vi "Merge_metadata.vi"(2 "New Value Priority high?":bool, 3 "Comments Row Number":i32, 4 "New Values In":string[](array[string]), 5 "New Chs In":string[](array[string]), 6 "Orig Values In":string[][](array[string]), 7 "Orig Chs In":string[](array[string])) -> (0 "Channel Values Out":string[][](array[string]), 1 "Ch names Out":string[](array[string]))   [LabVIEW 2010]
panel:
  out "Case":string
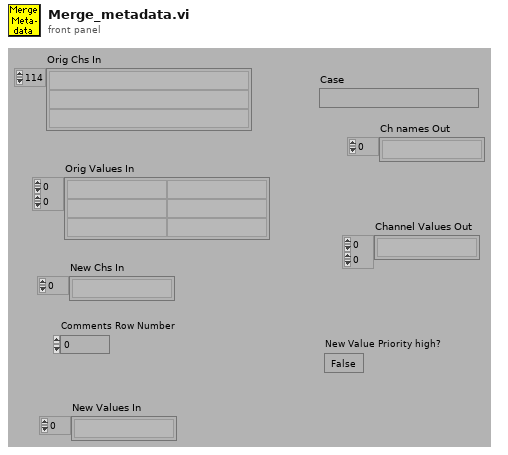
[diagram p1: front panel]
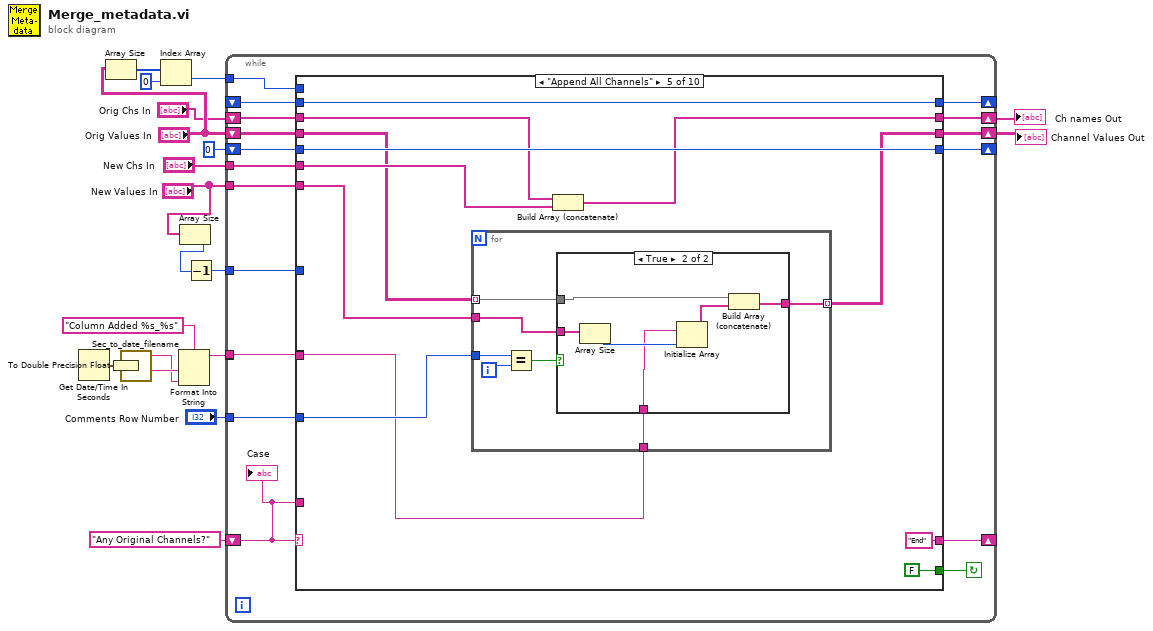
[diagram p0: block diagram]
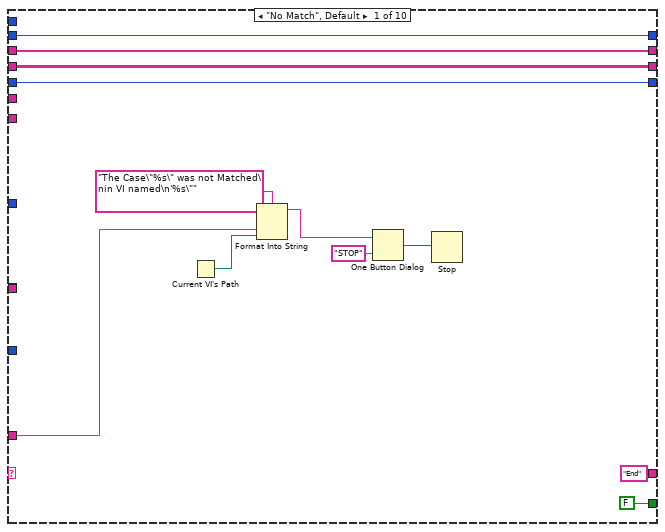
[diagram p2: hidden frame]
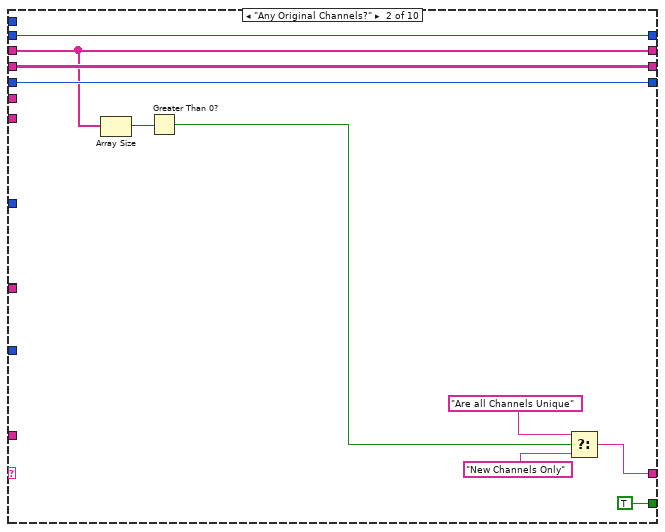
[diagram p3: hidden frame]
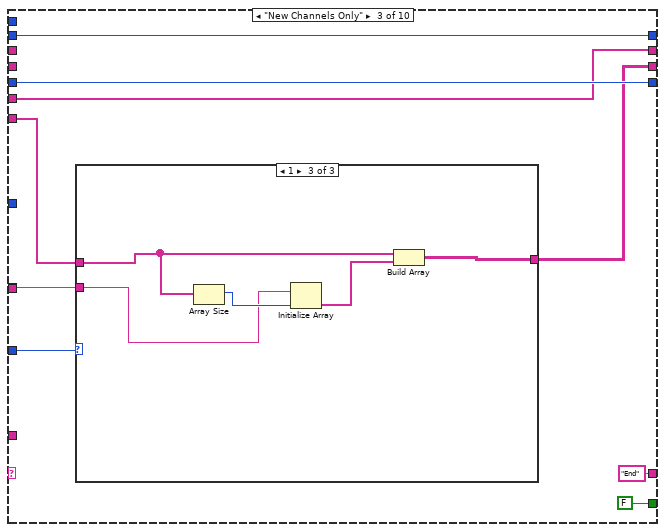
[diagram p4: hidden frame]
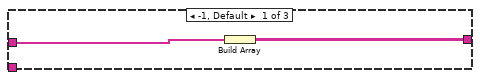
[diagram p5: hidden frame]
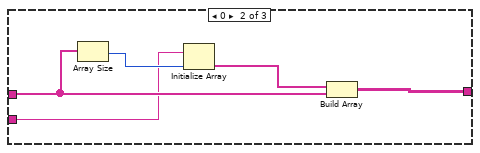
[diagram p6: hidden frame]
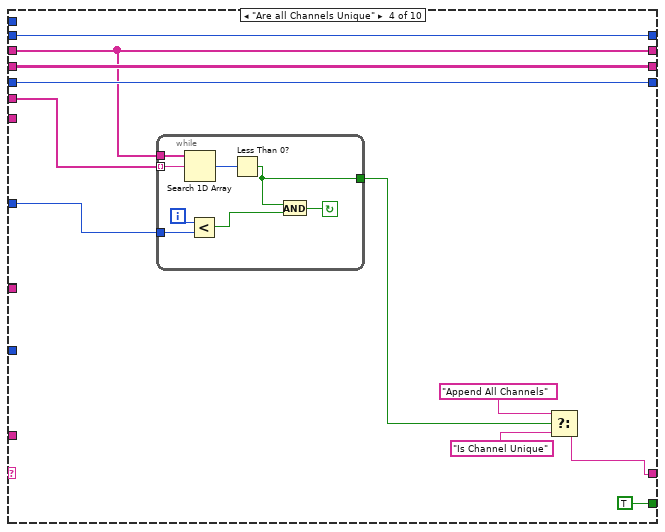
[diagram p7: hidden frame]
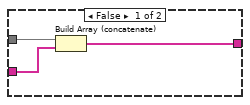
[diagram p8: hidden frame]
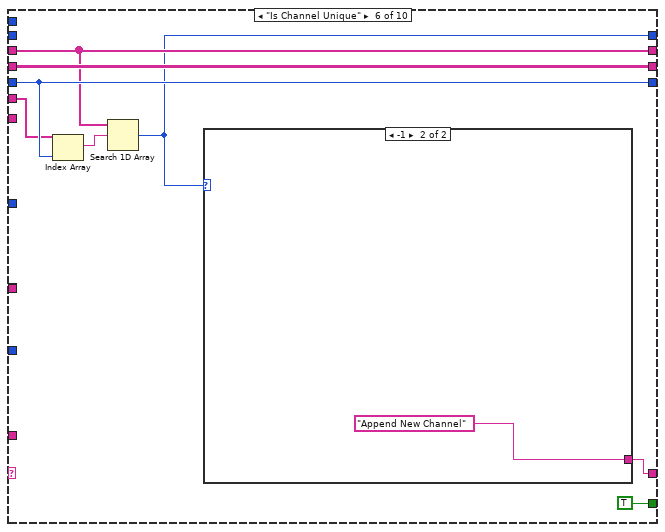
[diagram p9: hidden frame]
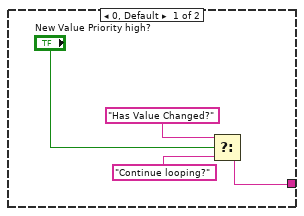
[diagram p10: hidden frame]
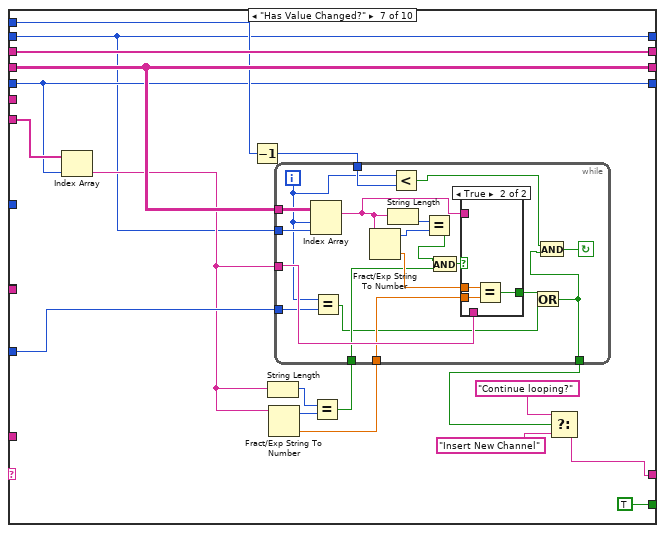
[diagram p11: hidden frame]
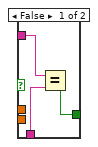
[diagram p12: hidden frame]
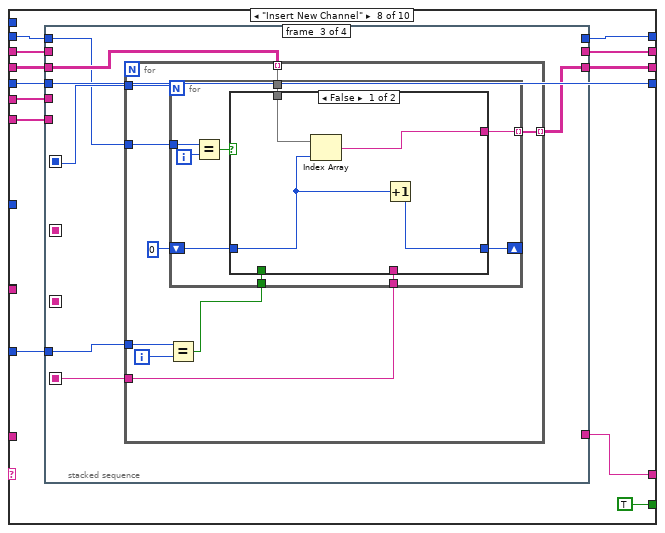
[diagram p13: hidden frame]
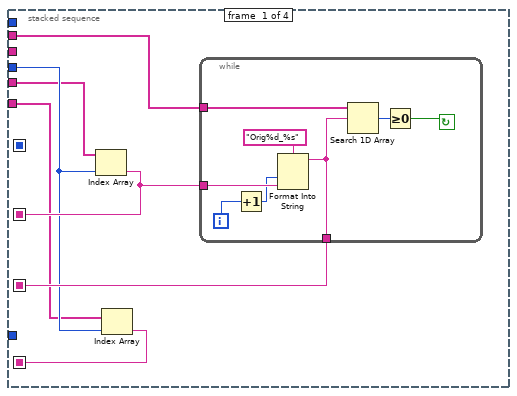
[diagram p14: hidden frame]
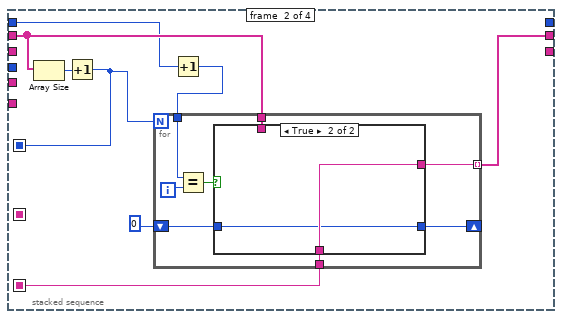
[diagram p15: hidden frame]
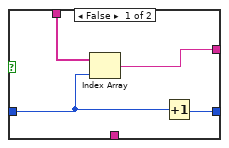
[diagram p16: hidden frame]
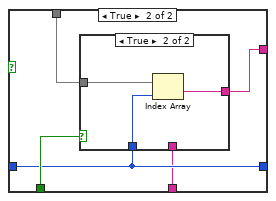
[diagram p17: hidden frame]
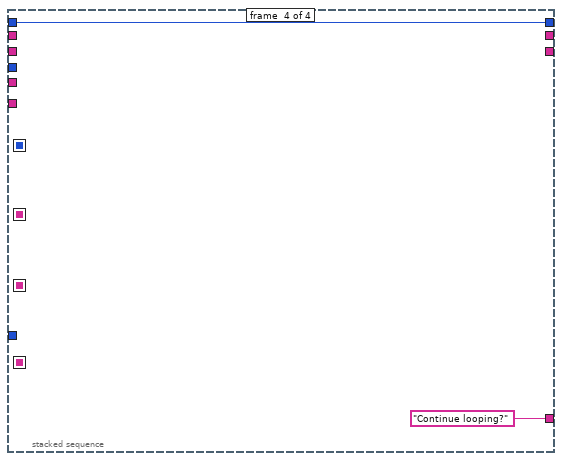
[diagram p19: hidden frame]
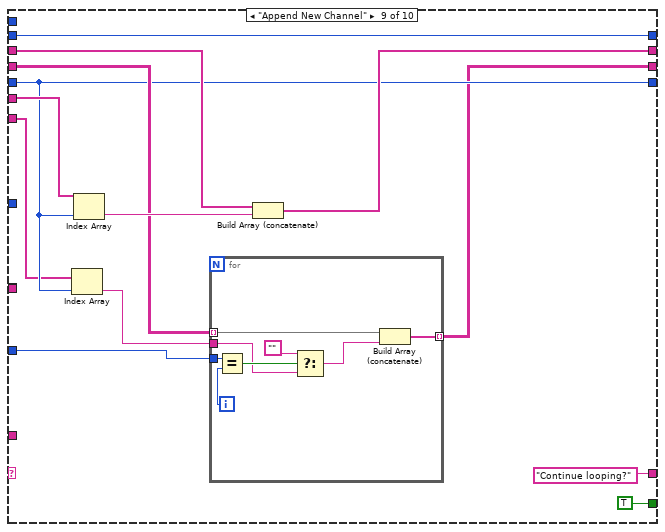
[diagram p20: hidden frame]
diagram:
  n1 = Get Date/Time In Seconds() -> (seconds since 1Jan1904=w1:timestamp)
  n2 = Array Size(array="Orig Values In") -> (size(s)=w14:i32[])
  n3 = To Double Precision Float(number=w1) -> (double precision float=w4:dbl)
  n4 = call "Sec_to_date_filename.vi"("seconds"=w4) -> ("Year"=w2:string, "Day"=w3:string)  [unwired: 2 out]
  n5 = Index Array(array=w14, index=0 ("Index")) -> (element=w11:i32)
  n6 = Format Into String(format string="Column Added %s_%s" ("Format String"), w3, w2) -> (resulting string=w5:string)  [unwired: 2 in, 1 out]
  n7 = Array Size(array="New Values In") -> (size(s)=w16:i32)
  n8 = Decrement(x=w16) -> (x-1=w15:i32)
  n9 = while {
    tunnel: w5 -> [w21]
    tunnel: w5 -> [w22]
    shift-left: _ -> [w24]
    shift-right: [w23] -> _
    tunnel: "Comments Row Number" -> [w25]
    tunnel: "New Values In" -> [w26]
    tunnel: "New Chs In" -> [w27]
    tunnel: w11 -> [w28]
    tunnel: w15 -> [w29]
    shift-left: 0 -> [w30]
    shift-right: [w31] -> _
    shift-left: "Orig Values In" -> [w33]
    shift-right: [w32] -> w18
    shift-left: "Orig Chs In" -> [w34]
    shift-right: [w35] -> w19
    shift-left: "Any Original Channels?" -> [w37]
    shift-right: [w36] -> _
    stop <- w38 continue-if-true
    n10 = case shown="\"Append All Channels\"" w37 {
      tunnel: [FALSE ("Results File?") TRUE ("Results File?") FALSE ("Results File?") TRUE ("Results File?") FALSE ("Results File?") TRUE ("Results File?") TRUE ("Results File?") TRUE ("Results File?") TRUE ("Results File?") w298] -> w38
      tunnel: w37 -> [w45 _ _ _ _ _ _ _ _ _]
      tunnel: w27 -> [_ _ w63 w85 w108 w129 _ w193 w284 _]
      tunnel: w26 -> [_ _ w62 _ w105 _ w156 w192 w278 _]
      tunnel: ["End" w55 "End" ("f") w91 "End" ("f") w135 w157 w188 "Continue looping?" "Is Channel Unique"] -> w36
      tunnel: [w42 w53 w63 w86 w107 w131 w159 w189 w281 w300] -> w35
      tunnel: w34 -> [w42 w53 _ w86 w109 w131 w159 w195 w282 w300]
      tunnel: w33 -> [w41 w59 _ w90 w106 w134 w155 w190 w280 w301]
      tunnel: [w41 w59 w65 w90 w104 w134 w155 w191 w276 w301] -> w32
      tunnel: [w40 w58 w68 w89 w111 w133 w143 w194 w279 w295] -> w31
      tunnel: w30 -> [w40 w58 w68 w89 w111 w133 w143 w194 w279 w296]
      tunnel: w29 -> [_ _ _ w84 _ _ _ _ _ w299]
      tunnel: w28 -> [_ _ _ _ _ _ w144 _ _ _]
      tunnel: w25 -> [_ _ w64 _ w103 _ w154 w187 w274 _]
      tunnel: w24 -> [w39 w57 w67 w82 w102 _ w142 w186 w273 w294]
      tunnel: [w39 w57 w67 w82 w102 w130 w142 w185 w273 w294] -> w23
      tunnel: w22 -> [_ _ w61 _ w101 _ _ _ _ _]
      tunnel: w21 -> [_ _ _ _ _ _ _ _ _ _]
      frame "No Match", Default {
        n11 = Current VI's Path() -> (path=w46:path)
        n12 = Format Into String(format string="The Case\"%s\" was not Matched\nin VI named\n'%s\"" ("Format String"), w45, w46) -> (resulting string=w49:string)  [unwired: 2 in, 1 out]
        n13 = One Button Dialog(message=w49, button name ("OK")="STOP") -> (true=w47:bool)
        n14 = Stop(stop? (T)=w47) -> ()
      }
      frame "Any Original Channels?" {
        n15 = Array Size(array=w53) -> (size(s)=w52:i32)
        n16 = Greater Than 0?(x=w52) -> (x > 0?=w51:bool)
        n17 = Select(t="Are all Channels Unique", s=w51, f="New Channels Only") -> (s? t:f=w55:string)
      }
      frame "New Channels Only" {
        n18 = case shown="1" w64 {
          tunnel: [w70 w76 w81] -> w65
          tunnel: w62 -> [w71 w75 w80]
          tunnel: w61 -> [_ w72 w77]
          frame -1, Default {
            n19 = Build Array(w71) -> (w70:string[][])
          }
          frame 0 {
            n20 = Array Size(array=w75) -> (size(s)=w74:i32)
            n21 = Initialize Array(w72, w74) -> (w73:string[])
            n22 = Build Array(w73, w75) -> (w76:string[][])
          }
          frame 1 {
            n23 = Array Size(array=w80) -> (size(s)=w79:i32)
            n24 = Initialize Array(w77, w79) -> (w78:string[])
            n25 = Build Array(w80, w78) -> (w81:string[][])
          }
        }
      }
      frame "Are all Channels Unique" {
        n26 = while {
          tunnel: [w93] -> w83
          tunnel: w84 -> [w96]
          tunnel: w85 -> [w99] mode=indexing
          tunnel: w86 -> [w100]
          i -> [w97]
          stop <- w94 continue-if-true
          n27 = Search 1D Array(1D array=w100, element=w99) -> (index of element=w98:i32)  [unwired: 1 out]
          n28 = Less?(x=w97, y=w96) -> (x < y?=w95:bool)
          n29 = Less Than 0?(x=w98) -> (x < 0?=w93:bool)
          n30 = And(x=w93, y=w95) -> (x .and. y?=w94:bool)
        }
        n31 = Select(t="Append All Channels" ("f"), s=w83, f="Is Channel Unique") -> (s? t:f=w91:string)
      }
      frame "Append All Channels" {
        n32 = for {
          tunnel: w106 -> [w119] mode=indexing
          tunnel: w105 -> [w118]
          tunnel: [w117] -> w104 mode=indexing
          tunnel: w103 -> [w115]
          tunnel: w101 -> [w113]
          i -> [w116]
          n33 = Equal?(x=w115, y=w116) -> (x = y?=w114:bool)
          n34 = case shown="True" w114 {
            tunnel: w119 -> [w122 w124]
            tunnel: w118 -> [w121 w128]
            tunnel: [w120 w123] -> w117
            tunnel: w113 -> [_ w126]
            frame False {
              n35 = Build Array (concatenate)(w122, w121) -> (w120:string[])
            }
            frame True {
              n36 = Array Size(array=w128) -> (size(s)=w127:i32)
              n37 = Initialize Array(w126, w127) -> (w125:string[])
              n38 = Build Array (concatenate)(w124, w125) -> (w123:string[])
            }
          }
        }
        n39 = Build Array (concatenate)(w109, w108) -> (w107:string[])
      }
      frame "Is Channel Unique" {
        n40 = Index Array(array=w129, index=w133) -> (element=w132:string)
        n41 = Search 1D Array(1D array=w131, element=w132) -> (index of element=w130:i32)  [unwired: 1 out]
        n42 = case shown="-1" w130 {
          tunnel: [w140 "Append New Channel"] -> w135
          frame 0, Default {
            n43 = Select(t="Has Value Changed?" ("f"), s="New Value Priority high?", f="Continue looping?") -> (s? t:f=w140:string)
          }
          frame -1 {
          }
        }
      }
      frame "Has Value Changed?" {
        n44 = Index Array(array=w156, index=w143) -> (element=w148:string)
        n45 = Decrement(x=w144) -> (x-1=w151:i32)
        n46 = String Length(string=w148) -> (length=w150:i32)
        n47 = Fract/Exp String To Number(string=w148) -> (offset past number=w149:i32, number=w146:dbl)  [unwired: 3 out]
        n48 = Equal?(x=w150, y=w149) -> (x = y?=w147:bool)
        n49 = while {
          tunnel: w154 -> [w161]
          tunnel: [w163] -> w145
          tunnel: w146 -> [w165]
          tunnel: w147 -> [w166]
          tunnel: w151 -> [w176]
          tunnel: w148 -> [w167]
          tunnel: w155 -> [w177]
          tunnel: w142 -> [w178]
          i -> [w162]
          stop <- w169 continue-if-true
          n50 = Index Array(array=w177, index (row)=w162, index (col)=w178) -> (element=w168:string)
          n51 = Equal?(x=w162, y=w161) -> (x = y?=w160:bool)
          n52 = Fract/Exp String To Number(string=w168) -> (offset past number=w174:i32, number=w171:dbl)  [unwired: 3 out]
          n53 = String Length(string=w168) -> (length=w175:i32)
          n54 = Less?(x=w162, y=w176) -> (x < y?=w170:bool)
          n55 = Equal?(x=w175, y=w174) -> (x = y?=w173:bool)
          n56 = And(x=w173, y=w166) -> (x .and. y?=w172:bool)
          n57 = case shown="True" w172 {
            tunnel: w171 -> [_ w184]
            tunnel: w165 -> [_ w183]
            tunnel: [w179 w182] -> w164
            tunnel: w168 -> [w181 _]
            tunnel: w167 -> [w180 _]
            frame False {
              n58 = Equal?(x=w181, y=w180) -> (x = y?=w179:bool)
            }
            frame True {
              n59 = Equal?(x=w184, y=w183) -> (x = y?=w182:bool)
            }
          }
          n60 = Or(x=w164, y=w160) -> (x .or. y?=w163:bool)
          n61 = And(x=w170, y=w163) -> (x .and. y?=w169:bool)
        }
        n62 = Select(t="Continue looping?", s=w145, f="Insert New Channel") -> (s? t:f=w157:string)
      }
      frame "Insert New Channel" {
        n63 = stacked-sequence {
          seq-local: [w202 _ _ _] -> [_ _ _ _]
          seq-local: [w201 _ _ _] -> [_ w214 _ _]
          seq-local: [w198 _ _ _] -> [_ _ w238 _]
          seq-local: [_ w216 _ _] -> [_ _ w236 _]
          tunnel: w195 -> [w203 w217 _ _]
          tunnel: w194 -> [w200 _ _ _]
          tunnel: w193 -> [w197 _ _ _]
          tunnel: w192 -> [w199 _ _ _]
          tunnel: [_ _ w239 _] -> w191
          tunnel: w190 -> [_ _ w237 _]
          tunnel: [_ w215 _ _] -> w189
          tunnel: [_ _ _ "Continue looping?"] -> w188
          tunnel: w187 -> [_ _ w235 _]
          tunnel: w186 -> [_ w213 w234 w271]
          tunnel: [_ _ _ w271] -> w185
          frame #0 {
            n64 = Index Array(array=w197, index=w200) -> (element=w202:string)
            n65 = Index Array(array=w199, index=w200) -> (element=w198:string)
            n66 = while {
              tunnel: [w204] -> w201
              tunnel: w202 -> [w210]
              tunnel: w203 -> [w211]
              i -> [w206]
              stop <- w207 continue-if-true
              n67 = Increment(x=w206) -> (x+1=w205:i32)
              n68 = Format Into String(format string="Orig%d_%s" ("Format String"), w205, w210) -> (resulting string=w204:string)  [unwired: 2 in, 1 out]
              n69 = Search 1D Array(1D array=w211, element=w204) -> (index of element=w208:i32)  [unwired: 1 out]
              n70 = Greater Or Equal To 0?(x=w208) -> (x >= 0?=w207:bool)
            }
          }
          frame #1 {
            n71 = Array Size(array=w217) -> (size(s)=w219:i32)
            n72 = Increment(x=w219) -> (x+1=w216:i32)
            n73 = Increment(x=w213) -> (x+1=w212:i32)
            n74 = for {
              N: w216 -> [_]
              shift-right: [w222] -> _
              shift-left: 0 -> [w223]
              tunnel: [w225] -> w215 mode=indexing
              tunnel: w214 -> [w224]
              tunnel: w217 -> [w221]
              tunnel: w212 -> [w220]
              i -> [w227]
              n75 = Equal?(x=w220, y=w227) -> (x = y?=w226:bool)
              n76 = case shown="True" w226 {
                tunnel: [w230 w233] -> w225
                tunnel: w224 -> [_ w233]
                tunnel: w221 -> [w231 _]
                tunnel: w223 -> [w229 w232]
                tunnel: [w228 w232] -> w222
                frame False {
                  n77 = Index Array(array=w231, index=w229) -> (element=w230:string)
                  n78 = Increment(x=w229) -> (x+1=w228:i32)
                }
                frame True {
                }
              }
            }
          }
          frame #2 {
            n79 = for {
              tunnel: w236 -> [w247]
              tunnel: w234 -> [w246]
              tunnel: [w245] -> w239 mode=indexing
              tunnel: w238 -> [w240]
              tunnel: w237 -> [w244] mode=indexing
              tunnel: w235 -> [w243]
              i -> [w242]
              n80 = Equal?(x=w243, y=w242) -> (x = y?=w241:bool)
              n81 = for {
                N: w247 -> [_]
                shift-right: [w251] -> _
                shift-left: 0 -> [w252]
                tunnel: w246 -> [w256]
                tunnel: [w254] -> w245 mode=indexing
                tunnel: w244 -> [w253]
                tunnel: w241 -> [w250]
                tunnel: w240 -> [w249]
                i -> [w257]
                n82 = Equal?(x=w256, y=w257) -> (x = y?=w255:bool)
                n83 = case shown="False" w255 {
                  tunnel: [w260 w263] -> w254
                  tunnel: w253 -> [w261 w264]
                  tunnel: w252 -> [w259 w265]
                  tunnel: [w258 w265] -> w251
                  tunnel: w250 -> [_ w266]
                  tunnel: w249 -> [_ w262]
                  frame False {
                    n84 = Index Array(array=w261, index=w259) -> (element=w260:string)
                    n85 = Increment(x=w259) -> (x+1=w258:i32)
                  }
                  frame True {
                    n86 = case shown="True" w266 {
                      tunnel: w265 -> [_ w270]
                      tunnel: w264 -> [_ w269]
                      tunnel: [w267 w268] -> w263
                      tunnel: w262 -> [w267 _]
                      frame False {
                      }
                      frame True {
                        n87 = Index Array(array=w269, index=w270) -> (element=w268:string)
                      }
                    }
                  }
                }
              }
            }
          }
          frame #3 {
          }
        }
      }
      frame "Append New Channel" {
        n88 = Index Array(array=w278, index=w279) -> (element=w277:string)
        n89 = Index Array(array=w284, index=w279) -> (element=w283:string)
        n90 = for {
          tunnel: w280 -> [w293] mode=indexing
          tunnel: w277 -> [w288]
          tunnel: [w292] -> w276 mode=indexing
          tunnel: w274 -> [w290]
          i -> [w291]
          n91 = Equal?(x=w290, y=w291) -> (x = y?=w289:bool)
          n92 = Select(t="", s=w289, f=w288) -> (s? t:f=w286:string)
          n93 = Build Array (concatenate)(w293, w286) -> (w292:string[])
        }
        n94 = Build Array (concatenate)(w282, w283) -> (w281:string[])
      }
      frame "Continue looping?" {
        n95 = Less?(x=w296, y=w299) -> (x < y?=w298:bool)
        n96 = Increment(x=w296) -> (x+1=w295:i32)
      }
    }
    "Case" <- w37
  }
  "Channel Values Out" <- w18
  "Ch names Out" <- w19
